vi "Get Font List.vi"(8 "Error In":errorcluster) -> (0 "Error Out":errorcluster, 4 "Font Array":string[](array[string]))   [LabVIEW 2012, in "Hover Button.xctl"]
doc: "This vi gets a list of all installed fonts on the computer so the user will be able to select on for the Boolean Text in the button. Currently, it works only for Windows machines."
uses:
  Hover Button.xctl
  <vilib>/registry/registry.llb/Registry RtKey.ctl
panel:
  # "This vi gets a list of all installed fonts on the computer so the user will be able to select on for the Boolean Text in the button"
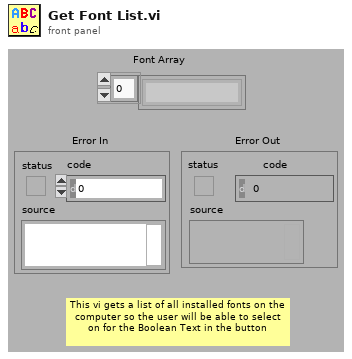
[diagram p1: front panel]
types:
  T1 = typedef "Registry RtKey.ctl" = enum32{"HKEY_CLASSES_ROOT", "HKEY_CURRENT_USER", "HKEY_LOCAL_MACHINE", "HKEY_USERS", "HKEY_PERFORMANCE_DATA", "HKEY_CURRENT_CONFIG", "HKEY_DYN_DATA"}
  T2 = typedef "Registry refnum.ctl" = refnum<k1>
  T3 = cluster{"numValues":i32, "maxValueNameLen":i32, "maxValueDataLen":i32}
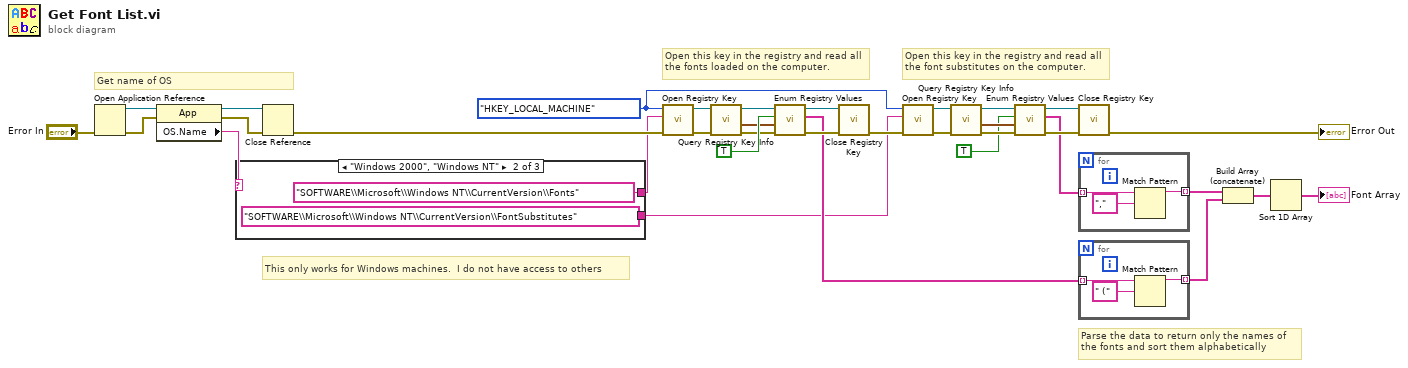
[diagram p0: block diagram]
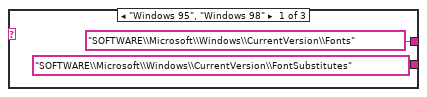
[diagram p2: hidden frame]
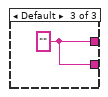
[diagram p3: hidden frame]
diagram:
  w11 = Registry_RtKey."HKEY_LOCAL_MACHINE" ("root key (HKEY_LOCAL_MACHINE)")
  # "Parse the data to return only the names of the fonts and sort them alphabetically"
  # "Get name of OS"
  # "Open this key in the registry and read all the font substitutes on the computer."
  # "Open this key in the registry and read all the fonts loaded on the computer."
  # "This only works for Windows machines.  I do not have access to others"
  n1 = Open Application Reference(8:"Error In") -> (0:w33:errorcluster, 3:w34:refnum<vi>)  [unwired: 3 in]
  n2 = property class="App"(reference=w34, error in=w33) -> (reference out=w32:refnum<vi>, error out=w31:errorcluster, "OS.Name"=w19:string)
  n3 = case shown="\"Windows 2000\", \"Windows NT\"" w19 {
    tunnel: ["SOFTWARE\\Microsoft\\Windows\\CurrentVersion\\Fonts" ("subkey") "SOFTWARE\\Microsoft\\Windows NT\\CurrentVersion\\Fonts" ("subkey") w39] -> w18
    tunnel: ["SOFTWARE\\Microsoft\\Windows\\CurrentVersion\\FontSubstitutes" ("subkey") "SOFTWARE\\Microsoft\\Windows NT\\CurrentVersion\\FontSubstitutes" ("subkey") w39] -> w6
    frame "Windows 95", "Windows 98" {
    }
    frame "Windows 2000", "Windows NT" {
    }
    frame Default {
      w39 = "" ("subkey")
    }
  }
  n4 = Close Reference(reference=w32, error in (no error)=w31) -> (error out=w22:errorcluster)
  n5 = call <vilib>:"Open Registry Key.vi"("error in (no error)"=w22, "subkey"=w18, "root key (HKEY_LOCAL_MACHINE)"=w11) -> ("error out"=w23:errorcluster, "refnum out"=w24:T2)  [unwired: 7 in]
  n6 = call <vilib>:"Query Registry Key Info.vi"("error in (no error)"=w23, "refnum"=w24) -> ("error out"=w27:errorcluster, "value info"=w26:T3, "refnum out"=w25:T2)  [unwired: 5 in, 2 out]
  n7 = call <vilib>:"Enum Registry Values.vi"("error in (no error)"=w27, "value info"=w26, "retrieve data? (F)"=TRUE, "refnum"=w25) -> ("error out"=w29:errorcluster, "values"=w21:string[], "refnum out"=w28:T2)  [unwired: 2 in, 3 out]
  n8 = call <vilib>:"Close Registry Key.vi"("error in (no error)"=w29, "refnum"=w28) -> ("error out"=w12:errorcluster)  [unwired: 5 in]
  n9 = call <vilib>:"Open Registry Key.vi"("error in (no error)"=w12, "subkey"=w6, "root key (HKEY_LOCAL_MACHINE)"=w11) -> ("error out"=w16:errorcluster, "refnum out"=w9:T2)  [unwired: 7 in]
  n10 = call <vilib>:"Query Registry Key Info.vi"("error in (no error)"=w16, "refnum"=w9) -> ("error out"=w14:errorcluster, "value info"=w15:T3, "refnum out"=w8:T2)  [unwired: 5 in, 2 out]
  n11 = call <vilib>:"Enum Registry Values.vi"("error in (no error)"=w14, "value info"=w15, "retrieve data? (F)"=TRUE, "refnum"=w8) -> ("error out"=w13:errorcluster, "values"=w5:string[], "refnum out"=w7:T2)  [unwired: 2 in, 3 out]
  n12 = call <vilib>:"Close Registry Key.vi"("error in (no error)"=w13, "refnum"=w7) -> ("error out"=→"Error Out":errorcluster)  [unwired: 5 in]
  n13 = for {
    tunnel: w5 -> [w41] mode=indexing
    tunnel: [w40] -> w4 mode=indexing
    n14 = Match Pattern(string=w41, regular expression=",") -> (before substring=w40:string)  [unwired: 1 in, 3 out]
  }
  n15 = for {
    tunnel: w21 -> [w44] mode=indexing
    tunnel: [w43] -> w2 mode=indexing
    n16 = Match Pattern(string=w44, regular expression=" (") -> (before substring=w43:string)  [unwired: 1 in, 3 out]
  }
  n17 = Build Array (concatenate)(w4, w2) -> (w3:string[])
  n18 = Sort 1D Array(array=w3) -> (sorted array=→"Font Array":string[])
